vi "SQLite Delete Balance Test.vi"(7 "Test DB Set Up Command":string, 8 "Error In (no error)":errorcluster, 11 "SQLite DB Operator In":refnum<class "SQLite DB Operator.lvclass">) -> (0 "Error Out":errorcluster, 3 "SQLite DB Operator Out":refnum<class "SQLite DB Operator.lvclass">)   [LabVIEW 2023]
uses:
  Clasess/SQLite DB Operator/SQLite DB Operator.lvclass
  Clasess/DB Records/Expenses Tracker Balance/Public/Ctrls/Balance.ctl
  Clasess/DB Records/Expenses Tracker Balance/Expenses Tracker Balance.lvclass
  H:/Desktop/LabVIEW/LabView Repo/Expenses-Tracker-DB-Operator/Interfaces/Expenses Tracker Record/Expenses Tracker Record.lvclass
  Support/Editing/Edit Record Assert Error.vi
  Support/Editing/Edit Record Assert Not Error.vi
  <vilib>/drjdpowell/SQLite Library/SQL Connection/Execute SQL (1D Cluster).vi
  <vilib>/addons/_JKI Toolkits/Caraya/classes/Assert/Assert Equal Value_Variant.vi
  <vilib>/addons/_JKI Toolkits/Caraya/classes/Test/Test.lvclass
  <vilib>/addons/_JKI Toolkits/Caraya/classes/Assert/Assert.lvclass
  <vilib>/drjdpowell/SQLite Library/SQLite.lvlib
  H:/Desktop/LabVIEW/LabView Repo/Expenses-Tracker-DB-Operator/Clasess/DB Records/Expenses Tracker Balance/Expenses Tracker Balance.lvclass
  <vilib>/drjdpowell/SQLite Library/SQL Connection/Connection.lvclass
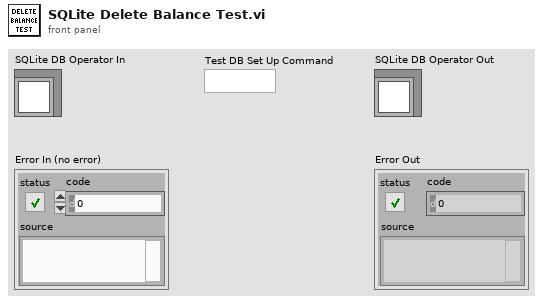
[diagram p1: front panel]
types:
  T1 = typedef "Expenses Tracker Balance.lvclass/Balance.ctl" = cluster{"ID":u8, "Value":dbl, "Last_update":timestamp}
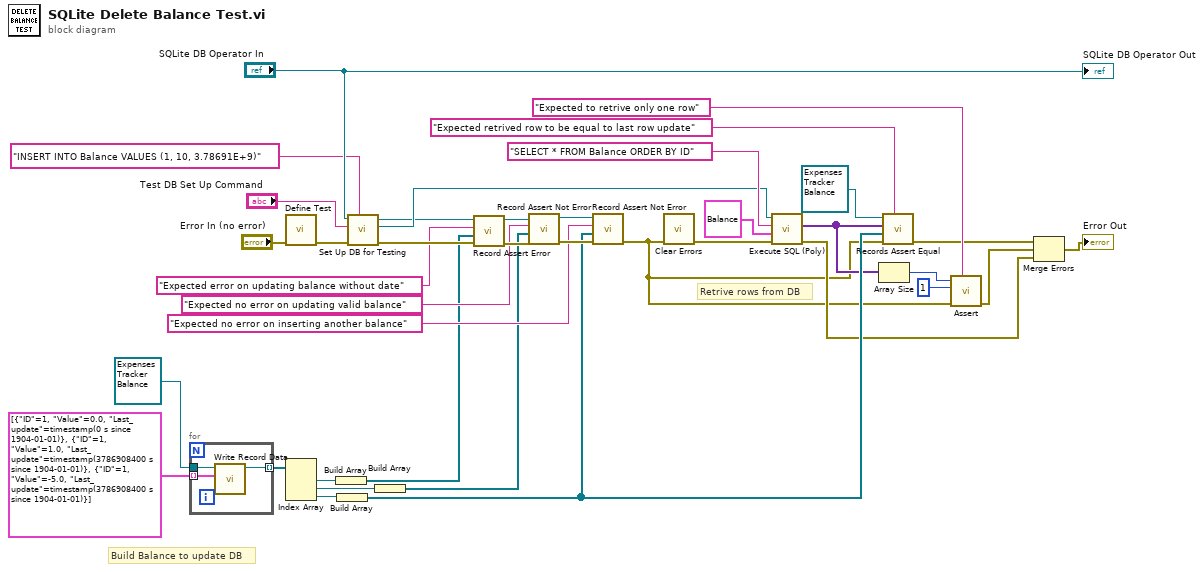
[diagram p0: block diagram]
diagram:
  # "Retrive rows from DB"
  # "Build Balance to update DB"
  n1 = for {
    tunnel: T1[] [{"ID"=1, "Value"=0.0, "Last_update"=timestamp(0 s since 1904-01-01)}, {"ID"=1, "Value"=1.0, "Last_update"=timestamp(3786908400 s since 1904-01-01)}, {"ID"=1, "Value"=-5.0, "Last_update"=timestamp(3786908400 s since 1904-01-01)}] ("Array") -> [w41] mode=indexing
    tunnel: refnum<class "Expenses Tracker Balance.lvclass"> refnum ("Expenses Tracker Category") -> [w40]
    tunnel: [w39] -> w35 mode=indexing
    n2 = call-dynamic "Write Record Data.vi"("Record"=w41, "Expenses Tracker Balance In"=w40) -> ("Expenses Tracker Balance Out"=w39:refnum<class "Expenses Tracker Balance.lvclass">)  [unwired: 8 in, 1 out]
  }
  n3 = call <vilib>:"Define Test.vi"("error in (no error)"="Error In (no error)") -> ("error out"=w25:errorcluster)  [unwired: 9 in, 1 out]
  n4 = Index Array(array=w35) -> (element #1=w34:refnum<class "Expenses Tracker Balance.lvclass">, element #2=w33:refnum<class "Expenses Tracker Balance.lvclass">, element #3=w30:refnum<class "Expenses Tracker Balance.lvclass">)  [unwired: 3 in]
  n5 = Build Array(w34) -> (w11:refnum<class "Expenses Tracker Balance.lvclass">[])
  n6 = Build Array(w30) -> (w9:refnum<class "Expenses Tracker Balance.lvclass">[])
  n7 = call "Set Up DB for Testing.vi"("Additional Set Up Commands"="INSERT INTO Balance VALUES (1, 10, 3.78691E+9)", "Error In (no error)"=w25, "Test DB Set Up Command"="Test DB Set Up Command", "SQLite DB Operator In"="SQLite DB Operator In") -> ("Error Out"=w19:errorcluster, "SQLite Connection"=w24:refnum<class "Connection.lvclass">, "SQLite DB Operator Out"=w15:refnum<class "SQLite DB Operator.lvclass">)  [unwired: 5 in]
  n8 = Build Array(w33) -> (w10:refnum<class "Expenses Tracker Balance.lvclass">[])
  n9 = call-poly "Record Assert Error.vi"("Error In"=w19, "Records"=w11, "Assertion Label"="Expected error on updating balance without date" ("Label (VI Title)"), "SQLite DB Operator In"=w15) -> ("Error Out"=w22:errorcluster, "SQLite DB Operator Out"=w23:refnum<class "SQLite DB Operator.lvclass">)  [unwired: 6 in]
  n10 = call-poly "Record Assert Not Error.vi"("Error In"=w22, "Records"=w10, "Assertion Label"="Expected no error on updating valid balance" ("Label (VI Title)"), "SQLite DB Operator In"=w23) -> ("Error Out"=w20:errorcluster, "SQLite DB Operator Out"=w21:refnum<class "SQLite DB Operator.lvclass">)  [unwired: 6 in]
  n11 = call-poly "Record Assert Not Error.vi"("Error In"=w20, "Records"=w9, "Assertion Label"="Expected no error on inserting another balance" ("Label (VI Title)"), "SQLite DB Operator In"=w21) -> ("Error Out"=w2:errorcluster)  [unwired: 6 in, 1 out]
  n12 = call <vilib>:"Clear Errors.vi"("error in (no error)"=w2) -> ("error out"=w7:errorcluster)  [unwired: 5 in, 1 out]
  n13 = call-poly <vilib>:"Execute SQL (Poly).vi"("error in (no error)"=w7, "Cluster (or Array of Clusters)"=T1 {"ID"=0, "Value"=0.0, "Last_update"=timestamp(0 s since 1904-01-01)} ("Balance"), "SQL"="SELECT * FROM Balance ORDER BY ID", "SQLite Connection in"=w24) -> ("error out"=w3:errorcluster, "Result Set (Array of Clusters)"=w6:variant[])  [unwired: 5 in, 1 out]
  n14 = Array Size(array=w6) -> (size(s)=w29:i32)
  n15 = call "Records Assert Equal.vi"("Assertion Label"="Expected retrived row to be equal to last row update" ("Label (VI Title)"), "Error In"=w2, "Correct Records"=w9, "Typedef Records"=w6, "Expenses Tracker Record In"=refnum<class "Expenses Tracker Balance.lvclass"> refnum ("Expenses Tracker Category")) -> ("Error Out"=w5:errorcluster)  [unwired: 6 in]
  n16 = call-poly <vilib>:"Assert.vi"("Label"="Expected to retrive only one row" ("Label (VI Title)"), "error in (no error)"=w2, "Y"=1, "X"=w29) -> ("error out"=w4:errorcluster)  [unwired: 6 in, 1 out]
  n17 = Merge Errors(w5, w4, w3) -> (→"Error Out":errorcluster)
  "SQLite DB Operator Out" <- "SQLite DB Operator In"
